vi "Teleop.vi"(10 "Match Info":T2={"Autonomous Elapsed Seconds"=0.0, "TeleOp Elapsed Seconds"=0.0, "Disabled Elapsed Seconds"=0.0, "Visited Autonomous"=FALSE, "Visited TeleOp"=FALSE, "Visited Disabled"=FALSE, "Autonomous Settings"={"Autonomous Style"=enum."Independent", "VI Refnum"=refnum}}, 11 "Call Context":T3) -> ()   [LabVIEW 2018]
doc: "This VI is called for each TeleOp packet received from the DS where the robot is not disabled. It is often used to read from the joysticks and update I/O or to update setpoints for timed control loops. It should complete and return within 20 milliseconds or it may miss DS packets."
uses:
  <vilib>/Rock Robotics/WPI/DriverStation/WPI_DriverStationDerivedRobotMode.ctl
  <vilib>/Rock Robotics/WPI/DriverStation/WPI_DriverStationMatch Info.ctl
  <vilib>/Rock Robotics/WPI/Solenoid/WPI_SolenoidValue.ctl
  <vilib>/Rock Robotics/WPI/Utilities/WPI_GetSetVariantRefNum.vi
  <vilib>/Rock Robotics/WPI/RobotDrive/WPI_RobotDriveMecanumDrive_Cartesian.vi
  <vilib>/Rock Robotics/WPI/RobotDrive/WPI_RobotDriveArcadeDrive_Standard(NoSaturation).vi
  <vilib>/Rock Robotics/WPI/Solenoid/WPI_SolenoidSetEnum.vi
panel:
  out "Rear Lift Solenoid Value 2":T1=enum."Forward"
  out "Rear Lift Pressed 2":dbl
  out "Front Lift Solenoid Value":T1=enum."Forward"
  out "Front Lift Pressed":dbl
  out "Back Lift B":bool
  out "Back Lift A":bool
  out "Front Lift B":bool
  out "Front Lift A":bool
  out "Modify Hoist":dbl
  out "Limit Switch":bool
  out "Suction Solenoid Value":T1
  out "Suction Button Pressed":dbl
  out "Tilt Solenoid Value":T1=enum."Forward"
  out "Tilt Button Pressed":dbl
  out "Y value 2":dbl
  out "Z value":dbl
  out "Y value":dbl
  out "X value":dbl
  out "Button 11\nSuction Push Out":bool
  out "Button 9\nSuction Off":bool
  out "Button 7\nSuction Pull In":bool
  out "Button 5\nTilt Up":bool
  out "Button 3\nTilt Down":bool
  # "Drive Control"
  # "Hoist Control"
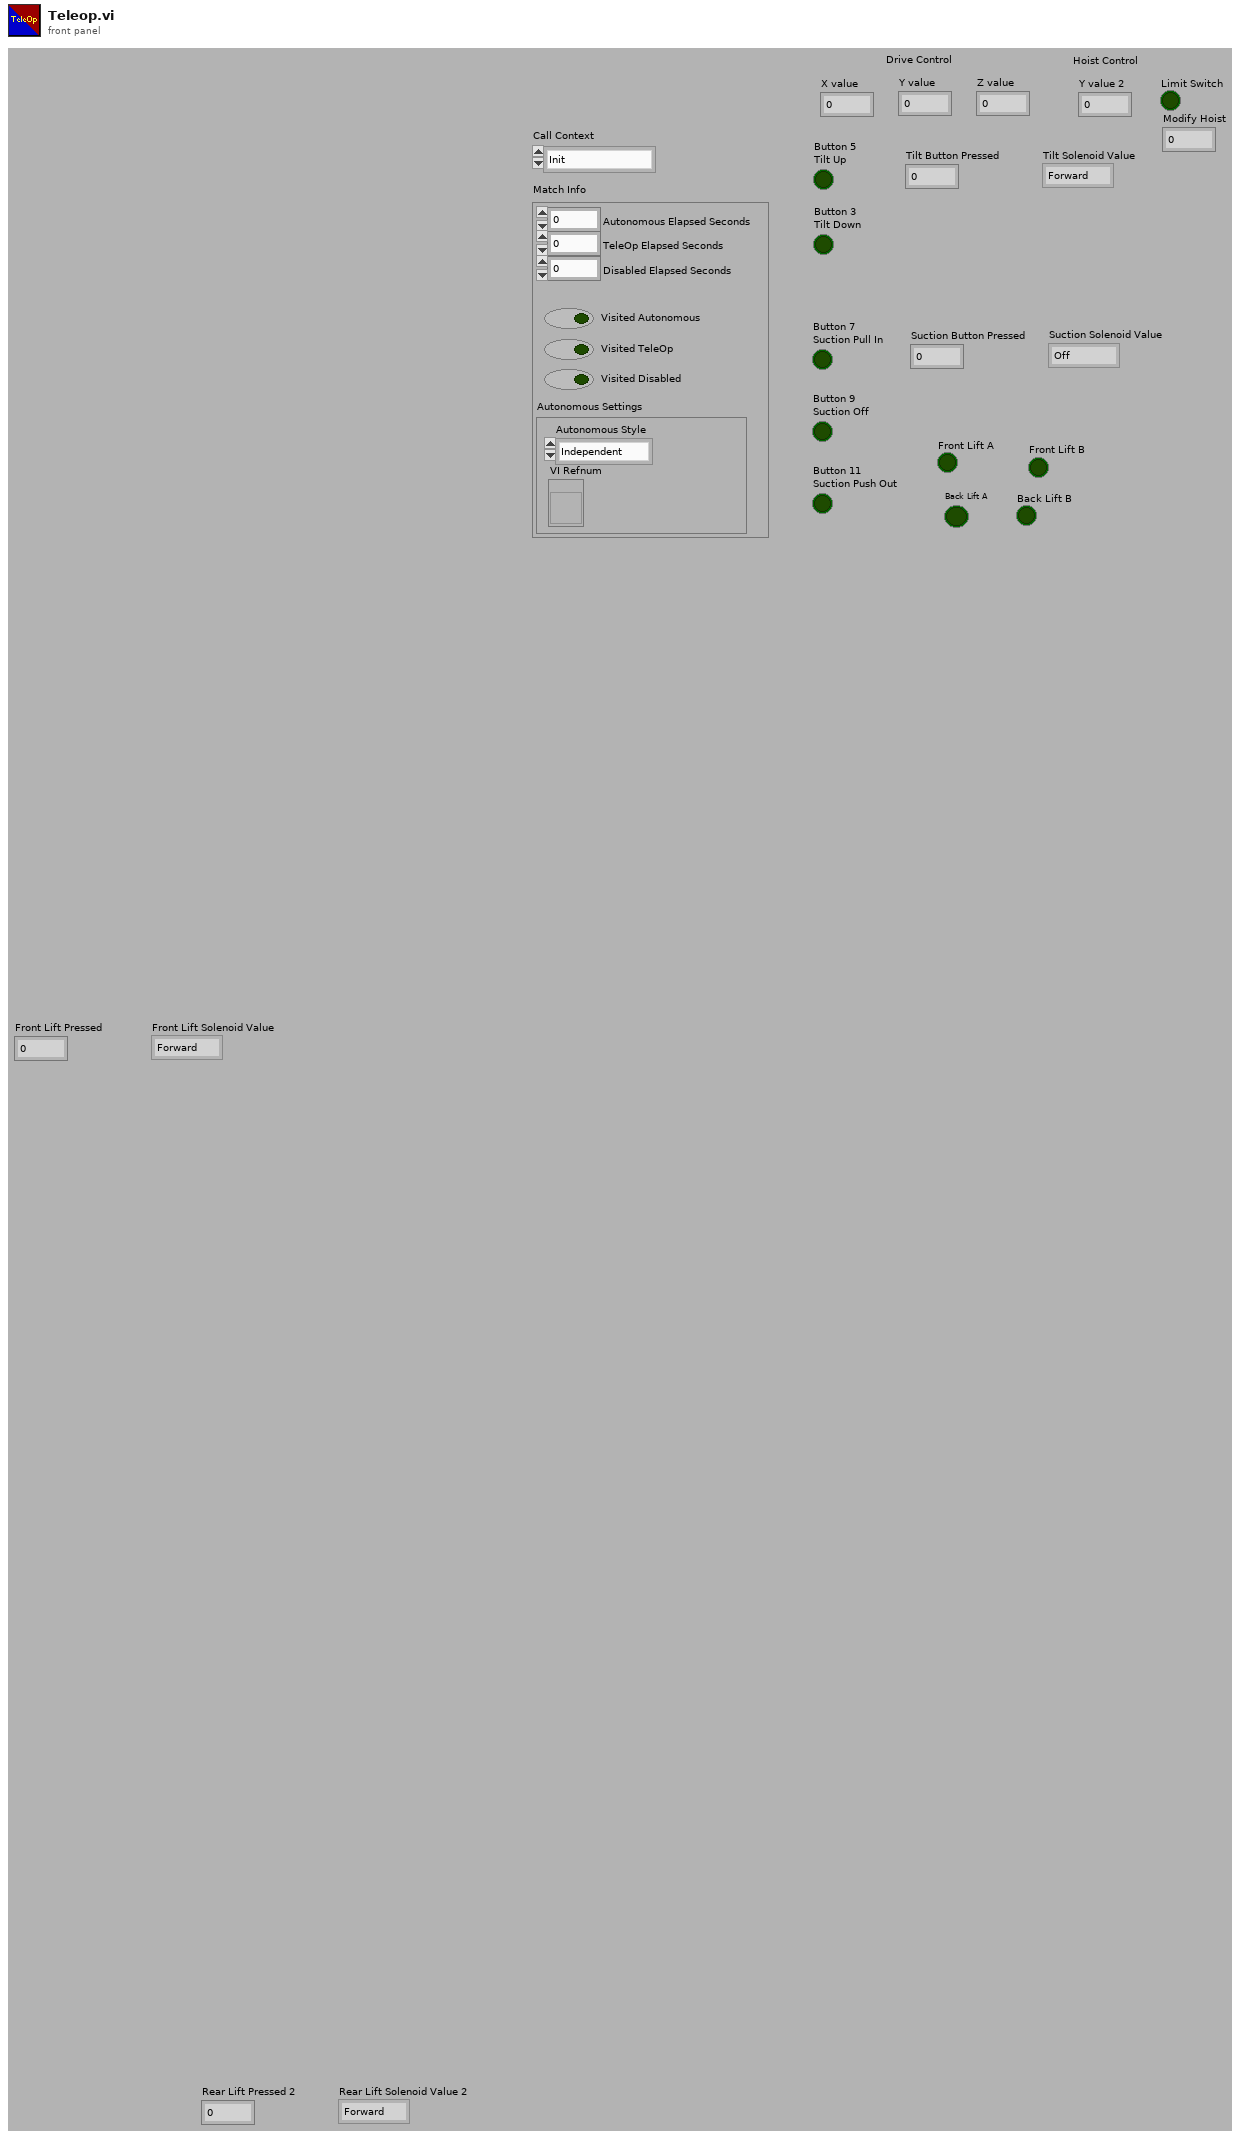
[diagram p1: front panel]
types:
  T1 = typedef "WPI_SolenoidValue.ctl" = enum16{"Off", "On", "Forward", "Reverse"}
  T2 = typedef "WPI_DriverStationMatch Info.ctl" = cluster{"Autonomous Elapsed Seconds":dbl, "TeleOp Elapsed Seconds":dbl, "Disabled Elapsed Seconds":dbl, "Visited Autonomous":bool, "Visited TeleOp":bool, "Visited Disabled":bool, "Autonomous Settings":cluster{"Autonomous Style":enum16{"Iterative", "Independent"}, "VI Refnum":refnum<vi>}}
  T3 = typedef "WPI_DriverStationDerivedRobotMode.ctl" = enum16{"Init", "Execute", "Stop"}
  T4 = typedef "WPI_DigitalInputDevRef.ctl" = cluster{"DevStatus":errorcluster, "DIO Channel":T5}
  T5 = typedef "FPGA_DIOChannel.ctl" = enum8{"DIO 0", "DIO 1", "DIO 2", "DIO 3", "DIO 4", "DIO 5", "DIO 6", "DIO 7", "DIO 8", "DIO 9", "DIO MXP 0", "DIO MXP 1", "DIO MXP 2", "DIO MXP 3", "DIO MXP 4", "DIO MXP 5", "DIO MXP 6", "DIO MXP 7", "DIO MXP 8", "DIO MXP 9", "DIO MXP 10", "DIO MXP 11", "DIO MXP 12", "DIO MXP 13", "DIO MXP 14", "DIO MXP 15", "SPI Port CS1", "SPI Port CS2", "SPI Port CS3", "SPI Port MISO", "SPI Port MOSI", "Invalid"}
  T6 = typedef "WPI_JoystickDevRef.ctl" = cluster{"Device":T7}
  T7 = typedef "WPI_JoystickDeviceEnum.ctl" = enum16{"USB 0", "USB 1", "USB 2", "USB 3", "USB 4", "USB 5"}
  T8 = typedef "WPI_RobotDriveDevRef.ctl" = cluster{"DevStatus":errorcluster, "Motors[]":T9[], "Square Inputs":bool, "Max Output":dbl}
  T9 = typedef "WPI_MotorControlDeviceRef.ctl" = cluster{"DeviceStatus":errorcluster, "Type":T10, "PWM":cluster{"PWM Channel":T11, "DeadBand":T12}, "CAN":cluster{"Device Number":u8, "SetOutput VI Ref":variant, "GetOutput VI Ref":variant, "Enable VI Ref":variant, "Disable VI Ref":variant, "Data":variant}, "Invert":bool, "DIO PWM":cluster{"PWM \"Enable\" Channel":T11, "DIOChannel":T5, "PWM Rate":dbl}}
  T10 = typedef "WPI_MotorControlType.ctl" = enum16{"PWM", "CAN", "DIO PWM"}
  T11 = typedef "FPGA_DIOPWMChannel.ctl" = enum8{"PWM 0", "PWM 1", "PWM 2", "PWM 3", "PWM 4", "PWM 5", "PWM 6", "PWM 7", "PWM 8", "PWM 9", "PWM MXP 0", "PWM MXP 1", "PWM MXP 2", "PWM MXP 3", "PWM MXP 4", "PWM MXP 5", "PWM MXP 6", "PWM MXP 7", "PWM MXP 8", "PWM MXP 9", "Invalid"}
  T12 = typedef "WPI_PWMDeadband.ctl" = cluster{"Name":string, "maxPositivePwm":i32, "minPositivePwm":i32, "centerPwm":i32, "maxNegativePwm":i32, "minNegativePwm":i32, "angularRange":u16}
  T13 = typedef "WPI_SolenoidDevRef.ctl" = cluster{"DevStatus":errorcluster, "Pneumatics Control Module":u8, "Forward Solenoid Channel":T14, "Reverse Solenoid Channel":T14}
  T14 = typedef "WPI_SolenoidChannel.ctl" = enum8{"Solenoid 0", "Solenoid 1", "Solenoid 2", "Solenoid 3", "Solenoid 4", "Solenoid 5", "Solenoid 6", "Solenoid 7", "Invalid"}
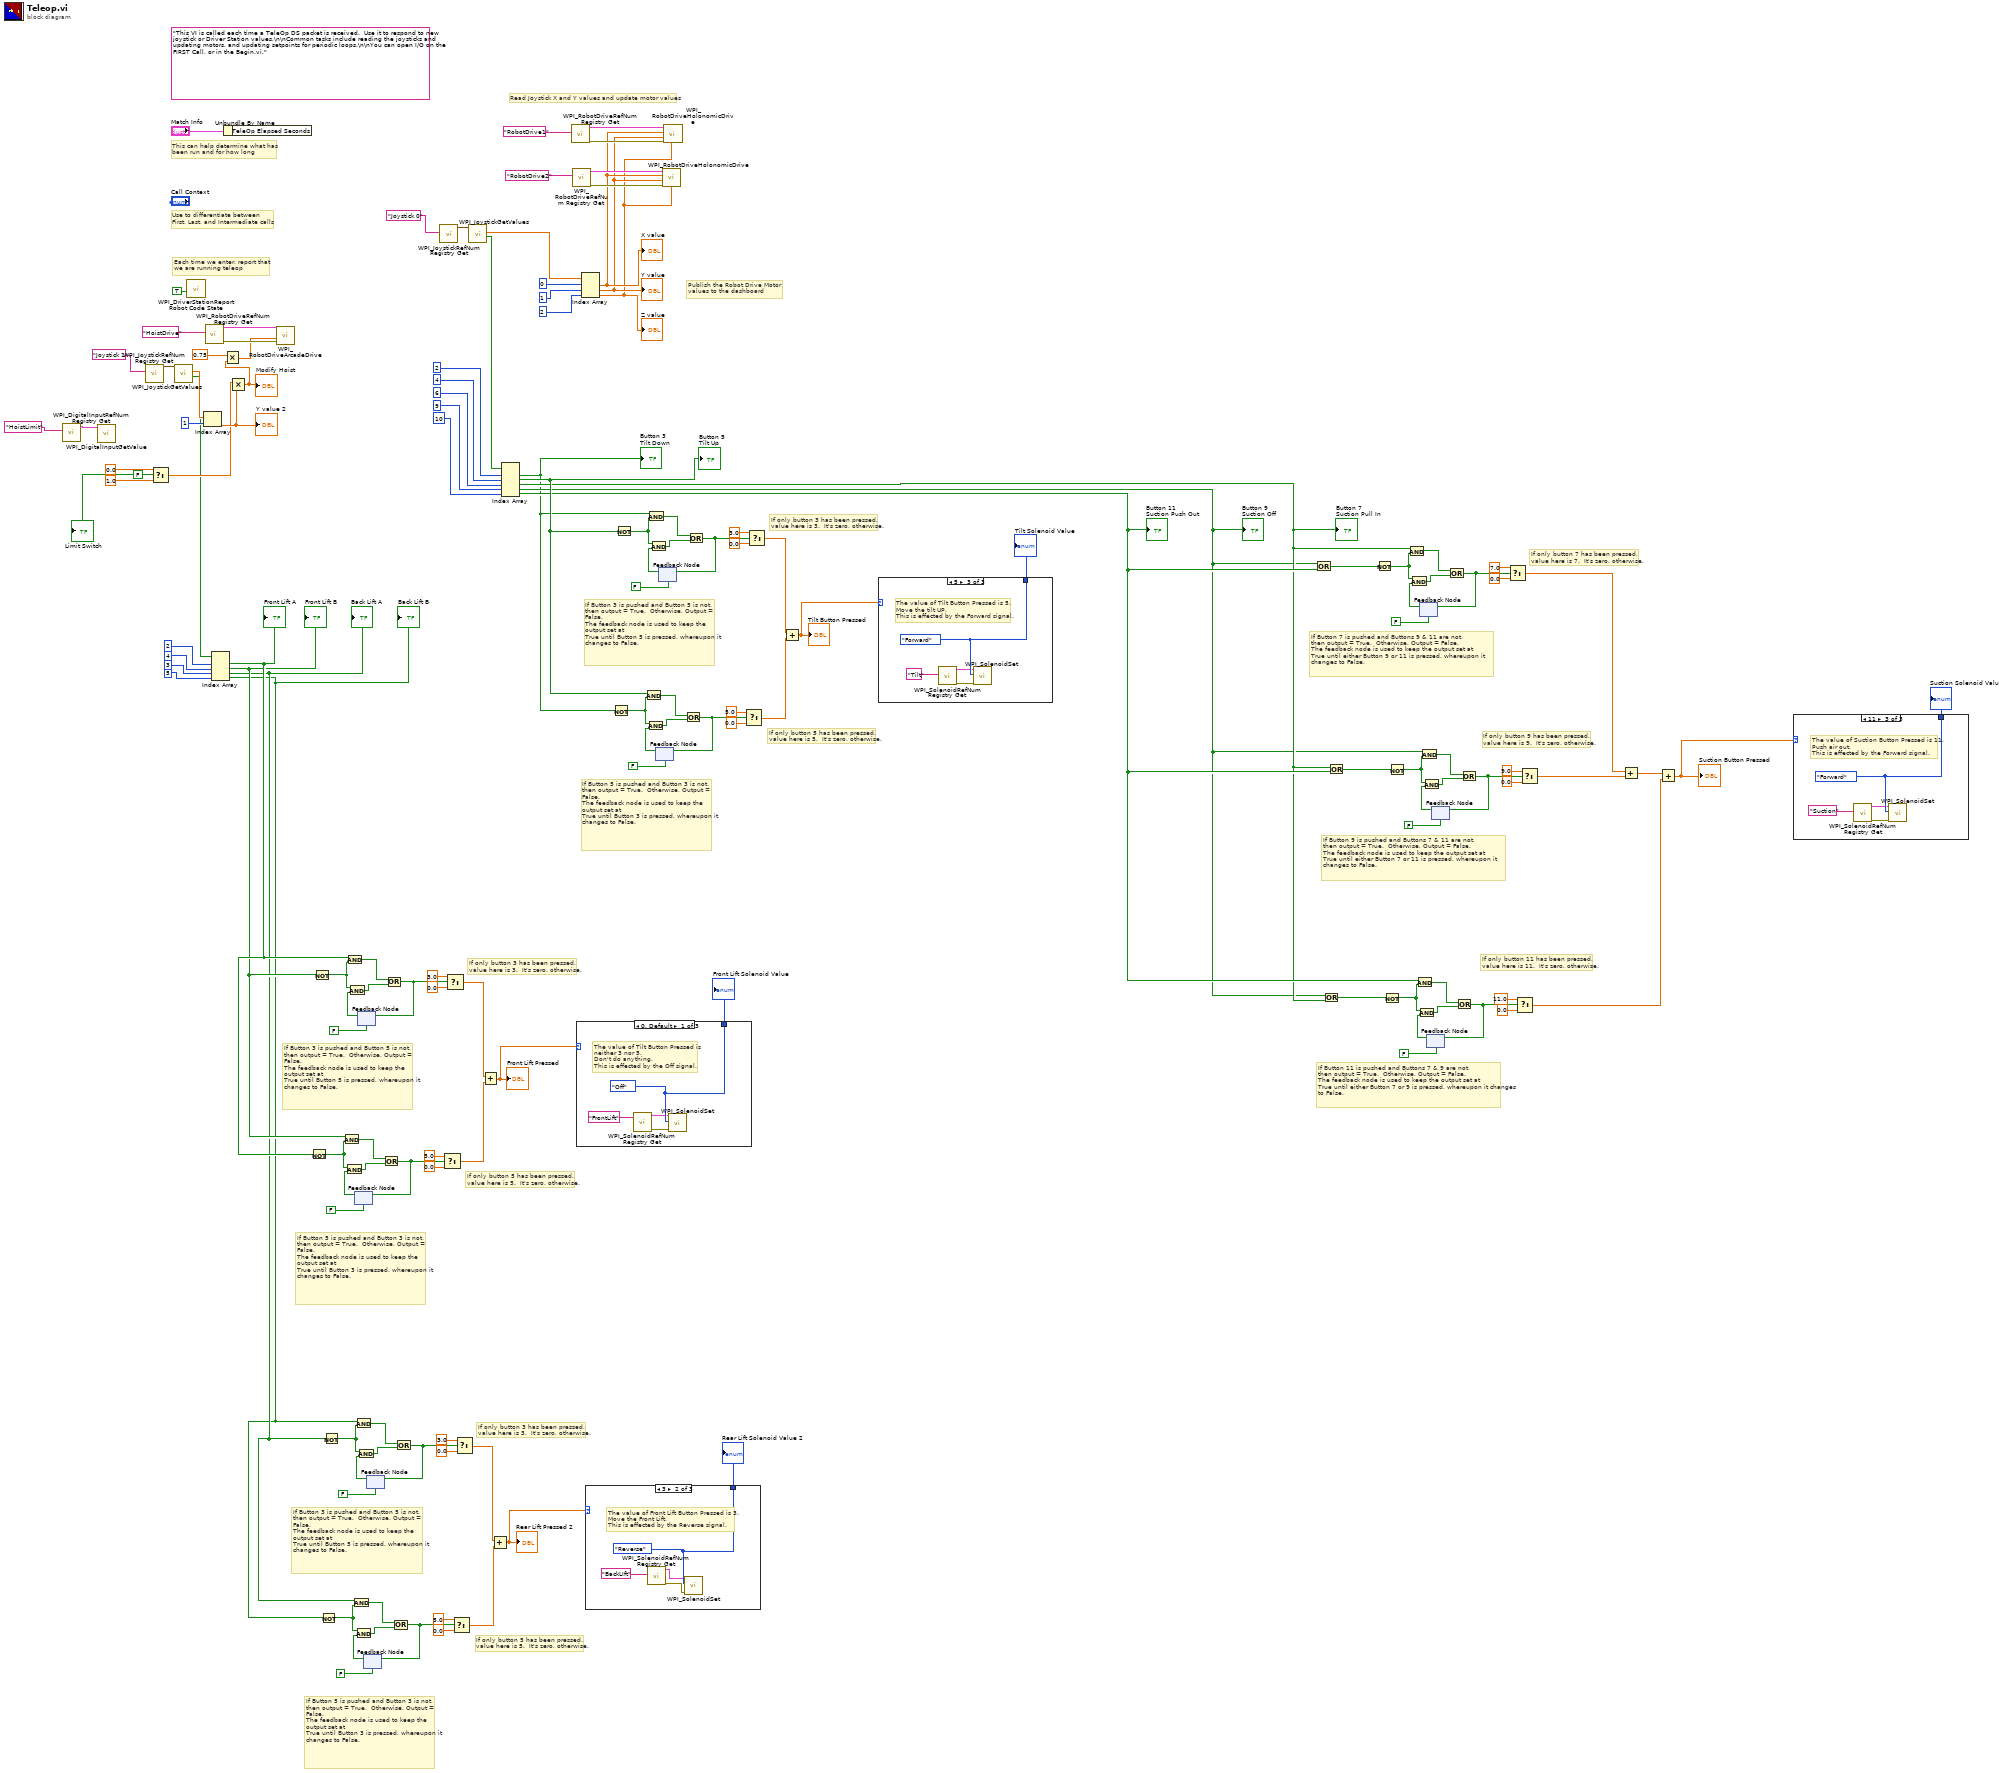
[diagram p0: block diagram]
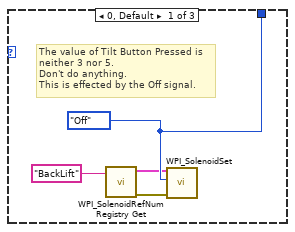
[diagram p2: hidden frame]
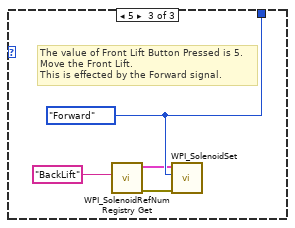
[diagram p3: hidden frame]
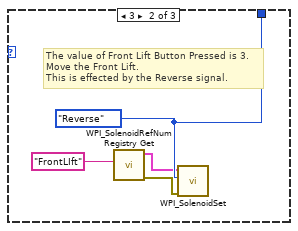
[diagram p4: hidden frame]
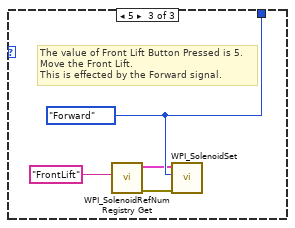
[diagram p5: hidden frame]
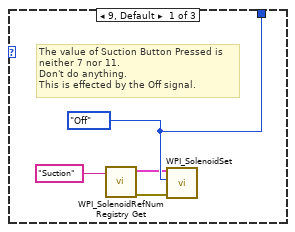
[diagram p6: hidden frame]
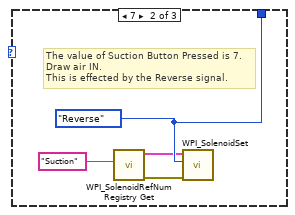
[diagram p7: hidden frame]
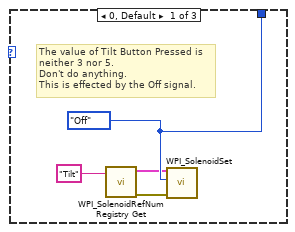
[diagram p8: hidden frame]
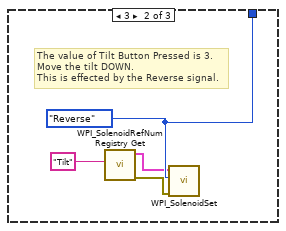
[diagram p9: hidden frame]
diagram:
  w53 = FALSE ("s")
  (unwired) "This VI is called each time a TeleOp DS packet is received.  Use it to respond to new joystick or Driver Station values.\n\nCommon tasks include reading the joysticks and updating motors, and updating setpoints for periodic loops.\n\nYou can open I/O on the FIRST Call, or in the Begin.vi."
  # "If only button 5 has been pressed,\nvalue here is 5.  It's zero, otherwise."
  # "If only button 3 has been pressed,\nvalue here is 3.  It's zero, otherwise."
  # "If Button 5 is pushed and Button 3 is not,\nthen output = True.  Otherwise, Output = False.\nThe feedback node is used to keep the output set at \nTrue until Button 3 is pressed, whereupon it changes to False."
  # "If Button 3 is pushed and Button 5 is not,\nthen output = True.  Otherwise, Output = False.\nThe feedback node is used to keep the output set at \nTrue until Button 5 is pressed, whereupon it changes to False."
  # "If only button 5 has been pressed,\nvalue here is 5.  It's zero, otherwise."
  # "If only button 3 has been pressed,\nvalue here is 3.  It's zero, otherwise."
  # "If Button 5 is pushed and Button 3 is not,\nthen output = True.  Otherwise, Output = False.\nThe feedback node is used to keep the output set at \nTrue until Button 3 is pressed, whereupon it changes to False."
  # "If Button 3 is pushed and Button 5 is not,\nthen output = True.  Otherwise, Output = False.\nThe feedback node is used to keep the output set at \nTrue until Button 5 is pressed, whereupon it changes to False."
  # "If only button 11 has been pressed,\nvalue here is 11.  It's zero, otherwise."
  # "If Button 11 is pushed and Buttons 7 & 9 are not,\nthen output = True.  Otherwise, Output = False.\nThe feedback node is used to keep the output set at \nTrue until either Button 7 or 9 is pressed, whereupon it changes to False."
  # "If only button 9 has been pressed,\nvalue here is 9.  It's zero, otherwise."
  # "If Button 9 is pushed and Buttons 7 & 11 are not,\nthen output = True.  Otherwise, Output = False.\nThe feedback node is used to keep the output set at \nTrue until either Button 7 or 11 is pressed, whereupon it changes to False."
  # "If only button 7 has been pressed,\nvalue here is 7.  It's zero, otherwise."
  # "If Button 7 is pushed and Buttons 9 & 11 are not,\nthen output = True.  Otherwise, Output = False.\nThe feedback node is used to keep the output set at \nTrue until either Button 9 or 11 is pressed, whereupon it changes to False."
  # "If only button 5 has been pressed,\nvalue here is 5.  It's zero, otherwise."
  # "If only button 3 has been pressed,\nvalue here is 3.  It's zero, otherwise."
  # "If Button 5 is pushed and Button 3 is not,\nthen output = True.  Otherwise, Output = False.\nThe feedback node is used to keep the output set at \nTrue until Button 3 is pressed, whereupon it changes to False."
  # "If Button 3 is pushed and Button 5 is not,\nthen output = True.  Otherwise, Output = False.\nThe feedback node is used to keep the output set at \nTrue until Button 5 is pressed, whereupon it changes to False."
  # "Publish the Robot Drive Motor\nvalues to the dashboard"
  # "Each time we enter, report that\nwe are running teleop"
  # "Use to differentiate between\nFirst, Last, and Intermediate calls"
  # "This can help determine what has\nbeen run and for how long"
  # "Read Joystick X and Y values and update motor values"
  n1 = call <vilib>:"WPI_DigitalInputRefNum Registry Get.vi"("refnum name"="HoistLimit") -> ("DigitalInputDevRef"=w54:T4)  [unwired: 9 in, 1 out]
  n2 = call <vilib>:"WPI_DigitalInputGetValue.vi"("DigitalInputDevRef"=w54) -> ()  [unwired: 8 in, 3 out]
  n3 = call <vilib>:"WPI_JoystickRefNum Registry Get.vi"("refnum name"="Joystick 1") -> ("JoystickDevRef"=w132:T6)  [unwired: 1 in, 9 out]
  n4 = Select(t=0.0, s=w53, f=1.0) -> (s? t:f=w58:dbl)
  n5 = call <vilib>:"WPI_JoystickGetValues.vi"("JoystickDevRef"=w132) -> ("Buttons"=w50:bool[], "Axes"=w131:dbl[])  [unwired: 6 in, 3 out]
  n6 = call <vilib>:"WPI_DriverStationReport Robot Code State.vi"("TeleOp"=TRUE ("Autonomous")) -> ()  [unwired: 10 in, 1 out]
  n7 = Index Array(array=w131, index=1) -> (element=w117:dbl)
  "Y value 2" <- w117
  n8 = call <vilib>:"WPI_RobotDriveRefNum Registry Get.vi"("refnum name"="HoistDrive") -> ("error out"=w118:errorcluster, "RobotDriveDevRef"=w119:T8)  [unwired: 9 in]
  n9 = Index Array(array=w50, index #1=2 ("index"), index #2=4 ("index"), index #3=3 ("index"), index #4=5 ("index")) -> (element #1=w27:bool, element #2=w26:bool, element #3=w5:bool, element #4=w4:bool)
  "Front Lift A" <- w27
  "Front Lift B" <- w26
  "Back Lift A" <- w5
  "Back Lift B" <- w4
  n10 = Unbundle By Name("Match Info") -> ()  [unwired: 1 out]
  n11 = Multiply(x=w58, y=w117) -> (x*y=w2:dbl)
  "Modify Hoist" <- w2
  n12 = Multiply(x=0.75, y=w2) -> (x*y=w1:dbl)
  n13 = call-poly <vilib>:"WPI_RobotDriveArcadeDrive.vi"("error in (no error)"=w118, "Y axis value"=w1, "RobotDriveDevRef"=w119) -> ()  [unwired: 6 in, 3 out]
  n14 = Not(x=w27) -> (.not. x?=w41:bool)
  n15 = Not(x=w26) -> (.not. x?=w47:bool)
  n16 = Not(x=w4) -> (.not. x?=w19:bool)
  n17 = Not(x=w5) -> (.not. x?=w25:bool)
  n18 = And(x=w26, y=w41) -> (x .and. y?=w40:bool)
  n19 = And(x=w27, y=w47) -> (x .and. y?=w46:bool)
  n20 = And(x=w5, y=w19) -> (x .and. y?=w18:bool)
  n21 = feedback #1(FALSE) -> (w38:bool)
  n22 = And(x=w41, y=w38) -> (x .and. y?=w39:bool)
  n23 = And(x=w4, y=w25) -> (x .and. y?=w24:bool)
  n24 = feedback #2(FALSE) -> (w44:bool)
  n25 = And(x=w47, y=w44) -> (x .and. y?=w45:bool)
  n26 = feedback #3(FALSE) -> (w16:bool)
  n27 = And(x=w19, y=w16) -> (x .and. y?=w17:bool)
  n28 = feedback #4(FALSE) -> (w22:bool)
  n29 = And(x=w25, y=w22) -> (x .and. y?=w23:bool)
  n30 = Or(x=w40, y=w39) -> (x .or. y?=w36:bool)
  n31 = feedback-in #1(w36) -> ()
  n32 = Or(x=w46, y=w45) -> (x .or. y?=w42:bool)
  n33 = feedback-in #2(w42) -> ()
  n34 = Or(x=w18, y=w17) -> (x .or. y?=w14:bool)
  n35 = feedback-in #3(w14) -> ()
  n36 = Or(x=w24, y=w23) -> (x .or. y?=w20:bool)
  n37 = feedback-in #4(w20) -> ()
  n38 = call <vilib>:"WPI_JoystickRefNum Registry Get.vi"("refnum name"="Joystick 0") -> ("JoystickDevRef"=w145:T6)  [unwired: 1 in, 9 out]
  n39 = Select(t=5.0, s=w36, f=0.0) -> (s? t:f=w30:dbl)
  n40 = Select(t=3.0, s=w42, f=0.0) -> (s? t:f=w31:dbl)
  n41 = Select(t=5.0, s=w14, f=0.0) -> (s? t:f=w8:dbl)
  n42 = Select(t=3.0, s=w20, f=0.0) -> (s? t:f=w9:dbl)
  n43 = call <vilib>:"WPI_JoystickGetValues.vi"("JoystickDevRef"=w145) -> ("Buttons"=w142:bool[], "Axes"=w143:dbl[])  [unwired: 6 in, 3 out]
  n44 = Add(x=w31, y=w30) -> (x+y=w29:dbl)
  "Front Lift Pressed" <- w29
  n45 = Add(x=w9, y=w8) -> (x+y=w7:dbl)
  "Rear Lift Pressed 2" <- w7
  n46 = Index Array(array=w142, index #1=2 ("index"), index #2=4 ("index"), index #3=6 ("index"), index #4=9 ("index"), index #5=10 ("index")) -> (element #1=w59:bool, element #2=w96:bool, element #3=w61:bool, element #4=w60:bool, element #5=w62:bool)
  "Button 3\nTilt Down" <- w59
  "Button 5\nTilt Up" <- w96
  "Button 7\nSuction Pull In" <- w61
  "Button 9\nSuction Off" <- w60
  "Button 11\nSuction Push Out" <- w62
  n47 = call <vilib>:"WPI_RobotDriveRefNum Registry Get.vi"("refnum name"="RobotDrive1") -> ("error out"=w127:errorcluster, "RobotDriveDevRef"=w128:T8)  [unwired: 9 in]
  n48 = call <vilib>:"WPI_RobotDriveRefNum Registry Get.vi"("refnum name"="RobotDrive2") -> ("error out"=w124:errorcluster, "RobotDriveDevRef"=w125:T8)  [unwired: 9 in]
  n49 = case shown="0, Default" w29 {
    tunnel: [w151 w155 w159] -> w28
    frame 0, Default {
      w151 = WPI_SolenoidValue."Off" ("Value")
      # "The value of Tilt Button Pressed is \nneither 3 nor 5.\nDon't do anything.\nThis is effected by the Off signal."
      n50 = call <vilib>:"WPI_SolenoidRefNum Registry Get.vi"("refnum name"="FrontLift") -> ("error out"=w150:errorcluster, "SolenoidDevRef"=w149:T13)  [unwired: 9 in]
      n51 = call-poly <vilib>:"WPI_SolenoidSet.vi"("error in (no error)"=w150, "Value"=w151, "SolenoidDevRef"=w149) -> ()  [unwired: 7 in, 2 out]
    }
    frame 3 {
      w155 = WPI_SolenoidValue."Reverse" ("Value")
      # "The value of Front Lift Button Pressed is 3.\nMove the Front Lift.\nThis is effected by the Reverse signal."
      n52 = call <vilib>:"WPI_SolenoidRefNum Registry Get.vi"("refnum name"="FrontLIft") -> ("error out"=w152:errorcluster, "SolenoidDevRef"=w153:T13)  [unwired: 9 in]
      n53 = call-poly <vilib>:"WPI_SolenoidSet.vi"("error in (no error)"=w152, "Value"=w155, "SolenoidDevRef"=w153) -> ()  [unwired: 7 in, 2 out]
    }
    frame 5 {
      w159 = WPI_SolenoidValue."Forward" ("Value")
      # "The value of Front Lift Button Pressed is 5.\nMove the Front Lift.\nThis is effected by the Forward signal."
      n54 = call <vilib>:"WPI_SolenoidRefNum Registry Get.vi"("refnum name"="FrontLift") -> ("error out"=w156:errorcluster, "SolenoidDevRef"=w157:T13)  [unwired: 9 in]
      n55 = call-poly <vilib>:"WPI_SolenoidSet.vi"("error in (no error)"=w156, "Value"=w159, "SolenoidDevRef"=w157) -> ()  [unwired: 7 in, 2 out]
    }
  }
  "Front Lift Solenoid Value" <- w28
  n56 = Index Array(array=w143, index #1=0 ("index"), index #2=1 ("index"), index #3=2 ("index")) -> (element #1=w123:dbl, element #2=w122:dbl, element #3=w121:dbl)
  "X value" <- w123
  "Y value" <- w122
  "Z value" <- w121
  n57 = case shown="3" w7 {
    tunnel: [w163 w167 w171] -> w6
    frame 0, Default {
      w163 = WPI_SolenoidValue."Off" ("Value")
      # "The value of Tilt Button Pressed is \nneither 3 nor 5.\nDon't do anything.\nThis is effected by the Off signal."
      n58 = call <vilib>:"WPI_SolenoidRefNum Registry Get.vi"("refnum name"="BackLift") -> ("error out"=w162:errorcluster, "SolenoidDevRef"=w161:T13)  [unwired: 9 in]
      n59 = call-poly <vilib>:"WPI_SolenoidSet.vi"("error in (no error)"=w162, "Value"=w163, "SolenoidDevRef"=w161) -> ()  [unwired: 7 in, 2 out]
    }
    frame 3 {
      w167 = WPI_SolenoidValue."Reverse" ("Value")
      # "The value of Front Lift Button Pressed is 3.\nMove the Front Lift.\nThis is effected by the Reverse signal."
      n60 = call <vilib>:"WPI_SolenoidRefNum Registry Get.vi"("refnum name"="BackLIft") -> ("error out"=w164:errorcluster, "SolenoidDevRef"=w165:T13)  [unwired: 9 in]
      n61 = call-poly <vilib>:"WPI_SolenoidSet.vi"("error in (no error)"=w164, "Value"=w167, "SolenoidDevRef"=w165) -> ()  [unwired: 7 in, 2 out]
    }
    frame 5 {
      w171 = WPI_SolenoidValue."Forward" ("Value")
      # "The value of Front Lift Button Pressed is 5.\nMove the Front Lift.\nThis is effected by the Forward signal."
      n62 = call <vilib>:"WPI_SolenoidRefNum Registry Get.vi"("refnum name"="BackLift") -> ("error out"=w168:errorcluster, "SolenoidDevRef"=w169:T13)  [unwired: 9 in]
      n63 = call-poly <vilib>:"WPI_SolenoidSet.vi"("error in (no error)"=w168, "Value"=w171, "SolenoidDevRef"=w169) -> ()  [unwired: 7 in, 2 out]
    }
  }
  "Rear Lift Solenoid Value 2" <- w6
  n64 = Not(x=w59) -> (.not. x?=w110:bool)
  n65 = Not(x=w96) -> (.not. x?=w116:bool)
  n66 = And(x=w96, y=w110) -> (x .and. y?=w109:bool)
  n67 = And(x=w59, y=w116) -> (x .and. y?=w115:bool)
  n68 = feedback #5(FALSE) -> (w107:bool)
  n69 = And(x=w110, y=w107) -> (x .and. y?=w108:bool)
  n70 = feedback #6(FALSE) -> (w113:bool)
  n71 = And(x=w116, y=w113) -> (x .and. y?=w114:bool)
  n72 = call-poly <vilib>:"WPI_RobotDriveHolonomicDrive.vi"("Rotation"=w121, "error in (no error)"=w124, "Y"=w122, "X"=w123, "RobotDriveDevRef"=w125) -> ()  [unwired: 4 in, 3 out]
  n73 = call-poly <vilib>:"WPI_RobotDriveHolonomicDrive.vi"("Rotation"=w121, "error in (no error)"=w127, "Y"=w122, "X"=w123, "RobotDriveDevRef"=w128) -> ()  [unwired: 4 in, 3 out]
  n74 = Or(x=w109, y=w108) -> (x .or. y?=w105:bool)
  n75 = feedback-in #5(w105) -> ()
  n76 = Or(x=w115, y=w114) -> (x .or. y?=w111:bool)
  n77 = feedback-in #6(w111) -> ()
  n78 = Select(t=5.0, s=w105, f=0.0) -> (s? t:f=w99:dbl)
  n79 = Select(t=3.0, s=w111, f=0.0) -> (s? t:f=w100:dbl)
  n80 = Add(x=w100, y=w99) -> (x+y=w98:dbl)
  "Tilt Button Pressed" <- w98
  n81 = case shown="5" w98 {
    tunnel: [w175 w179 w183] -> w97
    frame 0, Default {
      w175 = WPI_SolenoidValue."Off" ("Value")
      # "The value of Tilt Button Pressed is \nneither 3 nor 5.\nDon't do anything.\nThis is effected by the Off signal."
      n82 = call <vilib>:"WPI_SolenoidRefNum Registry Get.vi"("refnum name"="Tilt") -> ("error out"=w174:errorcluster, "SolenoidDevRef"=w173:T13)  [unwired: 9 in]
      n83 = call-poly <vilib>:"WPI_SolenoidSet.vi"("error in (no error)"=w174, "Value"=w175, "SolenoidDevRef"=w173) -> ()  [unwired: 7 in, 2 out]
    }
    frame 3 {
      w179 = WPI_SolenoidValue."Reverse" ("Value")
      # "The value of Tilt Button Pressed is 3.\nMove the tilt DOWN.\nThis is effected by the Reverse signal."
      n84 = call <vilib>:"WPI_SolenoidRefNum Registry Get.vi"("refnum name"="Tilt") -> ("error out"=w176:errorcluster, "SolenoidDevRef"=w177:T13)  [unwired: 9 in]
      n85 = call-poly <vilib>:"WPI_SolenoidSet.vi"("error in (no error)"=w176, "Value"=w179, "SolenoidDevRef"=w177) -> ()  [unwired: 7 in, 2 out]
    }
    frame 5 {
      w183 = WPI_SolenoidValue."Forward" ("Value")
      # "The value of Tilt Button Pressed is 5.\nMove the tilt UP.\nThis is effected by the Forward signal."
      n86 = call <vilib>:"WPI_SolenoidRefNum Registry Get.vi"("refnum name"="Tilt") -> ("error out"=w180:errorcluster, "SolenoidDevRef"=w181:T13)  [unwired: 9 in]
      n87 = call-poly <vilib>:"WPI_SolenoidSet.vi"("error in (no error)"=w180, "Value"=w183, "SolenoidDevRef"=w181) -> ()  [unwired: 7 in, 2 out]
    }
  }
  "Tilt Solenoid Value" <- w97
  n88 = Or(x=w60, y=w62) -> (x .or. y?=w86:bool)
  n89 = Or(x=w60, y=w61) -> (x .or. y?=w68:bool)
  n90 = Or(x=w61, y=w62) -> (x .or. y?=w77:bool)
  n91 = Not(x=w86) -> (.not. x?=w95:bool)
  n92 = Not(x=w68) -> (.not. x?=w76:bool)
  n93 = Not(x=w77) -> (.not. x?=w85:bool)
  n94 = And(x=w61, y=w95) -> (x .and. y?=w94:bool)
  n95 = And(x=w62, y=w76) -> (x .and. y?=w75:bool)
  n96 = feedback #7(FALSE) -> (w92:bool)
  n97 = And(x=w95, y=w92) -> (x .and. y?=w93:bool)
  n98 = And(x=w60, y=w85) -> (x .and. y?=w84:bool)
  n99 = feedback #8(FALSE) -> (w73:bool)
  n100 = And(x=w76, y=w73) -> (x .and. y?=w74:bool)
  n101 = feedback #9(FALSE) -> (w82:bool)
  n102 = And(x=w85, y=w82) -> (x .and. y?=w83:bool)
  n103 = Or(x=w94, y=w93) -> (x .or. y?=w90:bool)
  n104 = feedback-in #7(w90) -> ()
  n105 = Or(x=w75, y=w74) -> (x .or. y?=w71:bool)
  n106 = feedback-in #8(w71) -> ()
  n107 = Or(x=w84, y=w83) -> (x .or. y?=w80:bool)
  n108 = feedback-in #9(w80) -> ()
  n109 = Select(t=7.0, s=w90, f=0.0) -> (s? t:f=w87:dbl)
  n110 = Select(t=11.0, s=w71, f=0.0) -> (s? t:f=w65:dbl)
  n111 = Select(t=9.0, s=w80, f=0.0) -> (s? t:f=w67:dbl)
  n112 = Add(x=w87, y=w67) -> (x+y=w66:dbl)
  n113 = Add(x=w66, y=w65) -> (x+y=w64:dbl)
  "Suction Button Pressed" <- w64
  n114 = case shown="11" w64 {
    tunnel: [w187 w191 w195] -> w63
    frame 9, Default {
      w187 = WPI_SolenoidValue."Off" ("Value")
      # "The value of Suction Button Pressed is \nneither 7 nor 11.\nDon't do anything.\nThis is effected by the Off signal."
      n115 = call <vilib>:"WPI_SolenoidRefNum Registry Get.vi"("refnum name"="Suction") -> ("error out"=w186:errorcluster, "SolenoidDevRef"=w185:T13)  [unwired: 9 in]
      n116 = call-poly <vilib>:"WPI_SolenoidSet.vi"("error in (no error)"=w186, "Value"=w187, "SolenoidDevRef"=w185) -> ()  [unwired: 7 in, 2 out]
    }
    frame 7 {
      w191 = WPI_SolenoidValue."Reverse" ("Value")
      # "The value of Suction Button Pressed is 7.\nDraw air IN.\nThis is effected by the Reverse signal."
      n117 = call <vilib>:"WPI_SolenoidRefNum Registry Get.vi"("refnum name"="Suction") -> ("error out"=w188:errorcluster, "SolenoidDevRef"=w189:T13)  [unwired: 9 in]
      n118 = call-poly <vilib>:"WPI_SolenoidSet.vi"("error in (no error)"=w188, "Value"=w191, "SolenoidDevRef"=w189) -> ()  [unwired: 7 in, 2 out]
    }
    frame 11 {
      w195 = WPI_SolenoidValue."Forward" ("Value")
      # "The value of Suction Button Pressed is 11.\nPush air out.\nThis is effected by the Forward signal."
      n119 = call <vilib>:"WPI_SolenoidRefNum Registry Get.vi"("refnum name"="Suction") -> ("error out"=w192:errorcluster, "SolenoidDevRef"=w193:T13)  [unwired: 9 in]
      n120 = call-poly <vilib>:"WPI_SolenoidSet.vi"("error in (no error)"=w192, "Value"=w195, "SolenoidDevRef"=w193) -> ()  [unwired: 7 in, 2 out]
    }
  }
  "Suction Solenoid Value" <- w63
  "Limit Switch" <- w53
